vi "HPMT_View.vi"() -> ()   [LabVIEW 2016, in "HPMT_Views.lvlib"]
uses:
  HPMT_Views.lvlib
  Commands/Command Factory/Command Factory.lvclass
  User Events/User Events.lvclass
  User Events/User Events.lvclass/User Events.ctl
  Typedefs/CommandTypes.ctl
  Typedefs/StateTypes.ctl
  Typedefs/HPMT_Typedefs.lvlib
  Controller/Controller.lvclass
  Settings/Settings.lvclass
panel:
  in  "Tab Control":enum32{"Control"}(tab)
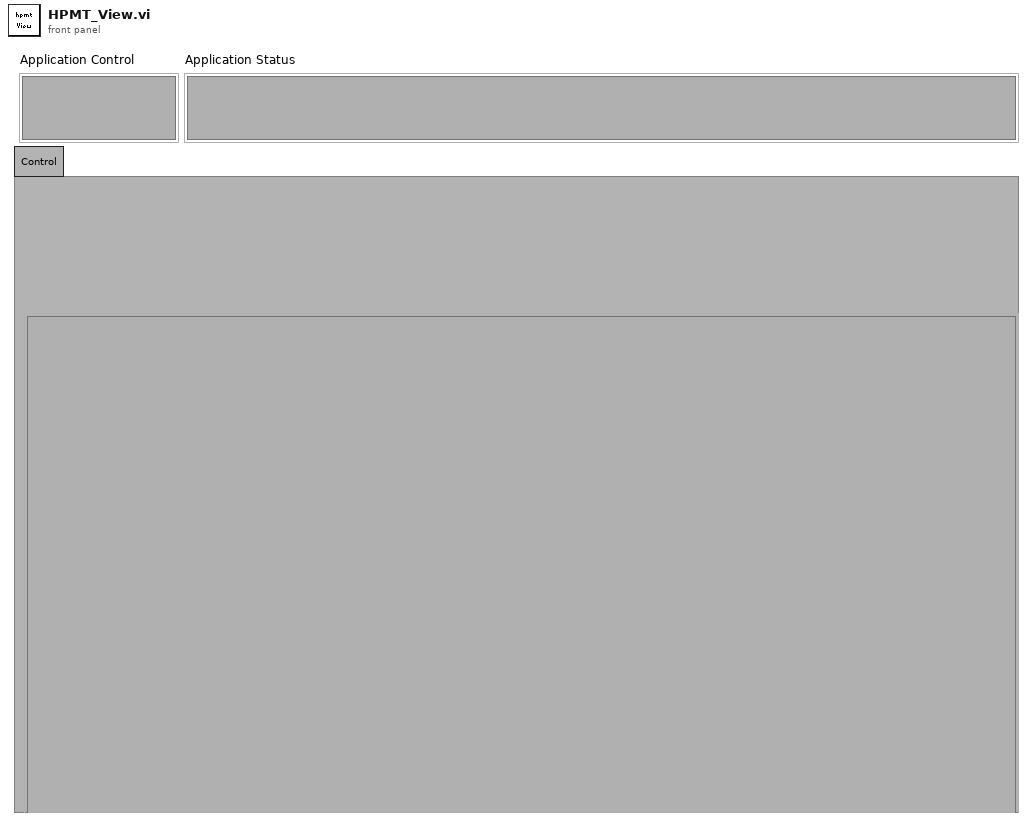
[diagram p1: front panel]
types:
  T1 = enum32{"invalid app kind", "Development System", "Run Time System", "Student Edition", "Embedded LabVIEW", "Evaluation", "Custom"}
  T2 = typedef "HPMT_Typedefs.lvlib/Publish Data Events.ctl" = cluster{"State":refnum<user-event>, "ErrorCode":refnum<user-event>, "Scan Progress":refnum<user-event>, "All Test Status":refnum<user-event>, "ActuatorData":refnum<user-event>, "Test Settings":refnum<user-event>, "Stop Constant Query":refnum<user-event>}
  T3 = typedef "HPMT_Typedefs.lvlib/Subscribe Data Events.ctl" = cluster{"Command":refnum<user-event>}
  T4 = cluster{"Event Registration Refnum":refnum<event-registration>, "Event Registration Refnum":refnum<event-registration>}
  T5 = typedef "HPMT_Typedefs.lvlib/CommandTypes.ctl" = enum16{"Start", "Enable", "Disable", "Standby", "Shutdown", "Update", "Stiffness", "Move Steps", "Constant Query", "Stop Constant Query"}
  T6 = typedef "HPMT_Typedefs.lvlib/StateTypes.ctl" = enum16{"Offline State", "Fault State", "Standby State", "Disabled State", "Enabled State", "Wait For User Input State", "Test Actuator State", "Manual State"}
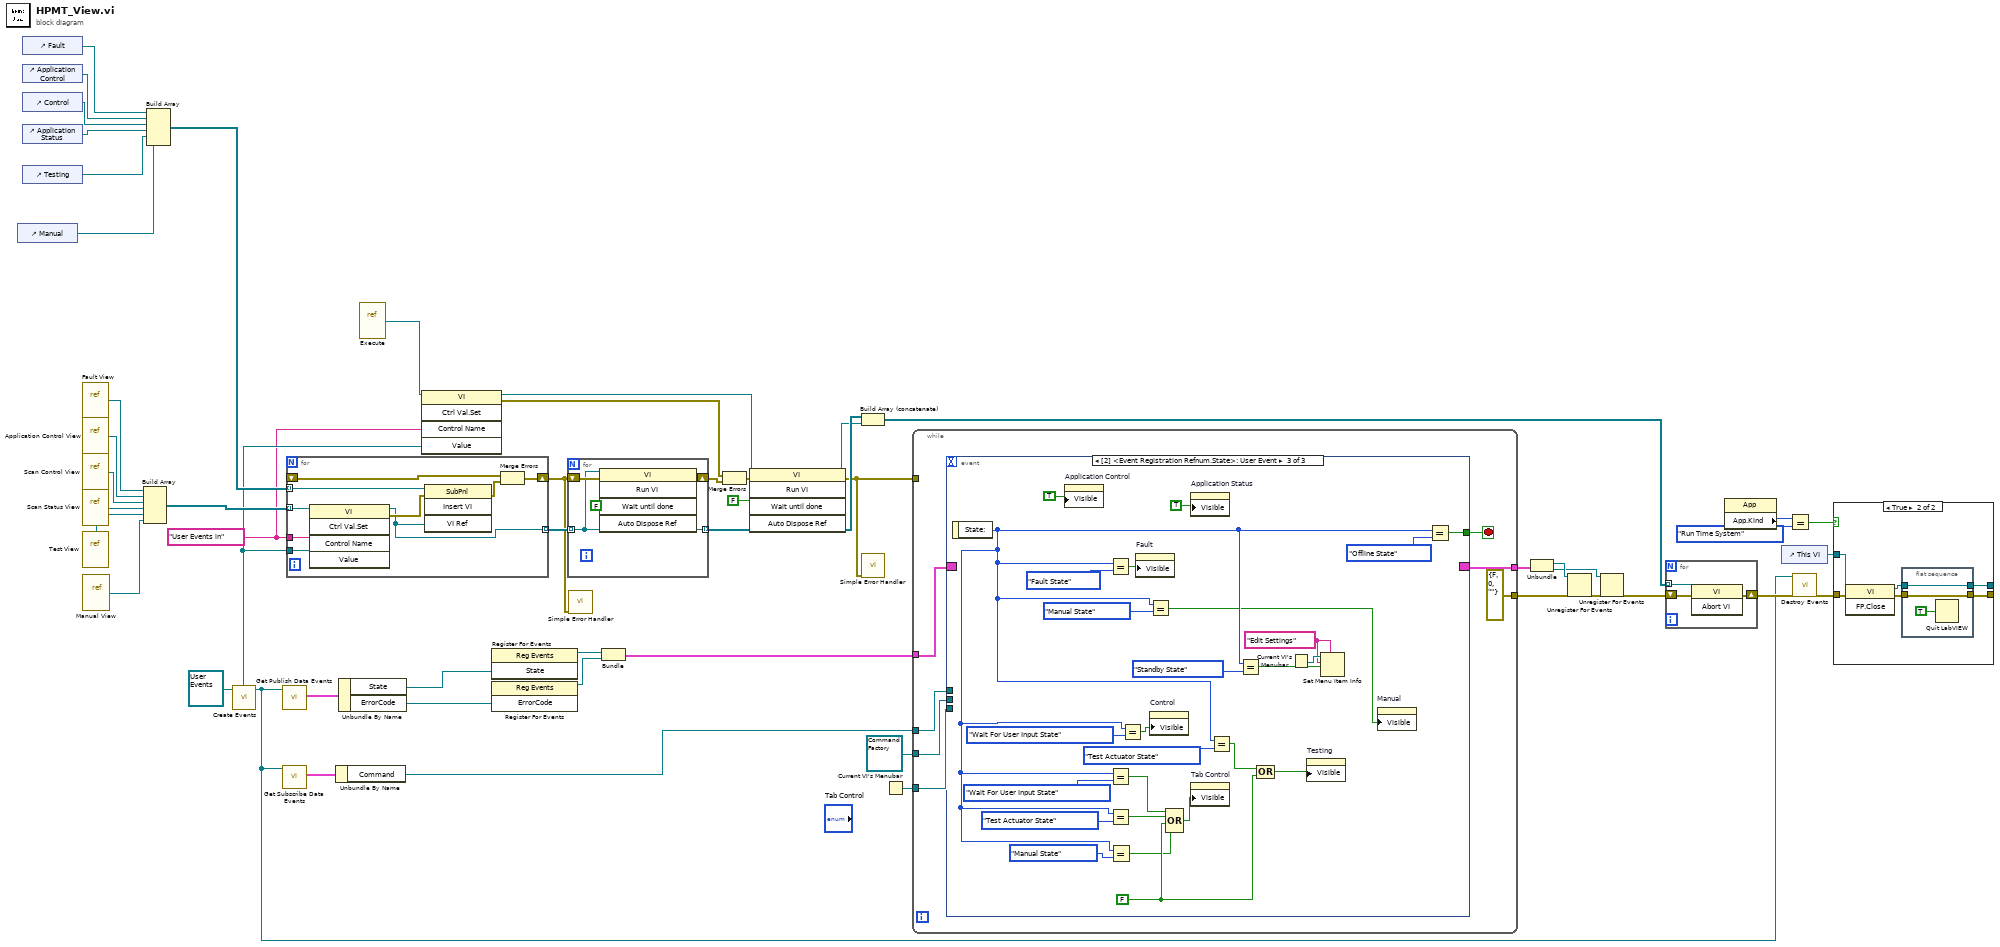
[diagram p0: block diagram]
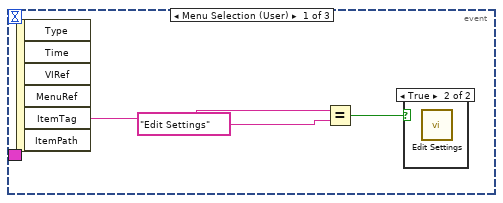
[diagram p3: hidden frame]
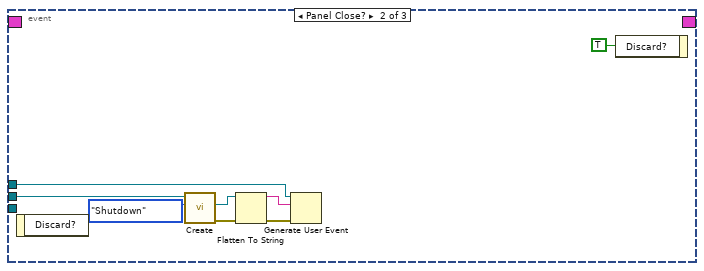
[diagram p5: hidden frame]
diagram:
  w21 = "User Events in" ("Control Name")
  n1 = control-ref of="Manual"() -> (w1:refnum<vi>)
  n2 = control-ref of="Fault"() -> (w11:refnum<vi>)
  n3 = control-ref of="Application Control"() -> (w10:refnum<vi>)
  n4 = control-ref of="Control"() -> (w9:refnum<vi>)
  n5 = control-ref of="Application Status"() -> (w8:refnum<vi>)
  n6 = control-ref of="Testing"() -> (w4:refnum<vi>)
  n7 = vi-ref "Fault View.vi"() -> (w26:refnum<vi>)
  n8 = vi-ref "Application Control View.vi"() -> (w7:refnum<vi>)
  n9 = vi-ref "Scan Control View.vi"() -> (w6:refnum<vi>)
  n10 = vi-ref "Scan Status View.vi"() -> (w12:refnum<vi>)
  n11 = vi-ref "Test View.vi"() -> (w3:refnum<vi>)
  n12 = vi-ref "Manual View.vi"() -> (w2:refnum<vi>)
  n13 = Build Array(w26, w7, w6, w12, w3, w2) -> (w24:refnum<vi>[])
  n14 = Build Array(w11, w10, w9, w8, w4, w1) -> (w25:refnum<vi>[])
  n15 = call "Create Events.vi"("UserEvents in"=refnum<class "User Events.lvclass"> refnum) -> ("UserEvents out"=w22:refnum<class "User Events.lvclass">)  [unwired: 9 in, 1 out]
  n16 = call "Get Publish Data Events.vi"("UserEvents in"=w22) -> ("Publish Data Events"=w46:T2)  [unwired: 9 in, 1 out]
  n17 = call "Get Subscribe Data Events.vi"("UserEvents in"=w22) -> ("Subscribe Data Events"=w44:T3)  [unwired: 9 in, 1 out]
  n18 = for {
    tunnel: w22 -> [w60]
    tunnel: w25 -> [w59] mode=indexing
    tunnel: w24 -> [w53] mode=indexing
    shift-right: [w58] -> w14
    shift-left: _ -> [w57]
    tunnel: [w52] -> w23 mode=indexing
    tunnel: w21 -> [w56]
    n19 = invoke class="VI" method="Ctrl Val.Set"(reference=w53, "Control Name"=w56, "Value"=w60) -> (reference out=w52:refnum<vi>, error out=w55:errorcluster)  [unwired: 2 in, 3 out]
    n20 = invoke on="Invoke Node" class="SubPnl" method="Insert VI"(reference=w59, error in=w55, "VI Ref"=w52) -> (error out=w54:errorcluster)  [unwired: 1 in, 3 out]
    n21 = Merge Errors(w57, w54) -> (w58:errorcluster)
  }
  n22 = Unbundle By Name(w44) -> ("Command"=w43:refnum<user-event>)
  n23 = Unbundle By Name(w46) -> ("State"=w42:refnum<user-event>, "ErrorCode"=w40:refnum<user-event>)
  n24 = vi-ref "Execute.vi"() -> (w37:refnum<vi>)
  n25 = invoke class="VI" method="Ctrl Val.Set"(reference=w37, "Control Name"=w21, "Value"=w22) -> (reference out=w36:refnum<vi>, error out=w18:errorcluster)  [unwired: 2 in, 3 out]
  n26 = register-events(w42) -> (reference out=w41:refnum<event-registration>)  [unwired: 2 in, 1 out]
  n27 = register-events(w40) -> (reference out=w39:refnum<event-registration>)  [unwired: 2 in, 1 out]
  n28 = for {
    shift-right: [w64] -> w20
    shift-left: w14 -> [w63]
    tunnel: w23 -> [w61] mode=indexing
    tunnel: [w61] -> w17 mode=indexing
    n29 = invoke class="VI" method="Run VI"(reference=w61, error in=w63, "Wait until done"=FALSE ("Wait Until Done")) -> (error out=w64:errorcluster)  [unwired: 2 in, 4 out]
  }
  n30 = call <vilib>:"Simple Error Handler.vi"("error in (no error)"=w14) -> ()  [unwired: 4 in, 5 out]
  n31 = Bundle("Event Registration Refnum"=w41, "Event Registration Refnum"=w39) -> (w34:T4)  [unwired: 1 in]
  n32 = Merge Errors(w18, w20) -> (w19:errorcluster)
  n33 = invoke class="VI" method="Run VI"(reference=w36, error in=w19, "Wait until done"=FALSE ("Wait Until Done")) -> (reference out=w16:refnum<vi>, error out=w13:errorcluster)  [unwired: 2 in, 3 out]
  n34 = Build Array (concatenate)(w17, w16) -> (w15:refnum<vi>[])
  n35 = call <vilib>:"Simple Error Handler.vi"("error in (no error)"=w13) -> ()  [unwired: 4 in, 5 out]
  n36 = Current VI's Menubar() -> (w47:refnum<k9>)
  n37 = while {
    tunnel: refnum<class "Command Factory.lvclass"> refnum ("CommandFactory.lvclass") -> [w68]
    tunnel: [errorcluster {"status"=FALSE, "code"=0, "source"=""} ("error out")] -> w35
    tunnel: w47 -> [w66]
    tunnel: w34 -> [w70]
    tunnel: w43 -> [w67]
    tunnel: [w65] -> w33
    tunnel: w13 -> [_]
    stop <- w69 stop-if-true
    n38 = event shown="[2] <Event Registration Refnum.State>: User Event" {
      selector: w70 -> [_ _ _]
      dyn-events: [_ _ _] -> w65
      timeout: _ -> [_ _ _]
      tunnel: [_ _ w107] -> w69
      tunnel: w68 -> [_ w79 _]
      tunnel: w67 -> [_ w76 _]
      tunnel: w66 -> [_ _ _]
      event Menu Selection (User) {
        n39 = event-data() -> ("ItemTag"=w72:string)  [unwired: 1 in, 5 out]
        n40 = Equal?(x=w72, y="Edit Settings") -> (x = y?=w74:bool)
        n41 = case shown="True" w74 {
          frame False {
          }
          frame True {
            n42 = call "Edit Settings.vi"() -> ()  [unwired: 10 in, 2 out]
          }
        }
      }
      event Panel Close? {
        n43 = event-data() -> ()  [unwired: 1 in, 1 out]
        n44 = call-dynamic "Create.vi"("Command Types"=CommandTypes."Shutdown" ("Command"), "Command Factory in"=w79) -> ("error out"=w82:errorcluster, "Command"=w81:refnum<class "Command.lvclass">)  [unwired: 7 in, 1 out]
        n45 = Flatten To String(anything=w81, error in (no error)=w82) -> (data string=w77:string, error out=w78:errorcluster)  [unwired: 2 in, 1 out]
        n46 = Generate User Event(user event=w76, event data cluster=w77, error in=w78) -> ()  [unwired: 1 in, 2 out]
        n47 = event-data("Discard?"=TRUE) -> ()  [unwired: 1 in, 1 out]
      }
      event User Event {
        w91 = FALSE
        w99 = "Edit Settings" ("menu tag")
        n48 = event-data() -> ("State:"=w84:T6)  [unwired: 1 in]
        n49 = property on="Application Control" class="SubPnl"("Visible"=TRUE) -> ()  [unwired: 2 in, 2 out]
        n50 = Equal?(x=w84, y=StateTypes."Fault State") -> (x = y?=w104:bool)
        n51 = Equal?(x=w84, y=StateTypes."Wait For User Input State") -> (x = y?=w94:bool)
        n52 = Equal?(x=w84, y=StateTypes."Test Actuator State") -> (x = y?=w88:bool)
        n53 = Equal?(x=w84, y=StateTypes."Manual State") -> (x = y?=w86:bool)
        n54 = Equal?(x=w84, y=StateTypes."Wait For User Input State") -> (x = y?=w89:bool)
        n55 = property on="Fault" class="SubPnl"("Visible"=w104) -> ()  [unwired: 2 in, 2 out]
        n56 = Equal?(x=w84, y=StateTypes."Manual State") -> (x = y?=w83:bool)
        n57 = property on="Control" class="SubPnl"("Visible"=w89) -> ()  [unwired: 2 in, 2 out]
        n58 = Compound Arithmetic op=OR(w94, w88, w91, w86) -> (w93:bool)
        n59 = property on="Application Status" class="SubPnl"("Visible"=TRUE) -> ()  [unwired: 2 in, 2 out]
        n60 = property on="Tab Control" class="TabCtl (strict)"("Visible"=w93) -> ()  [unwired: 2 in, 2 out]
        n61 = Equal?(x=w84, y=StateTypes."Test Actuator State") -> (x = y?=w92:bool)
        n62 = Equal?(x=w84, y=StateTypes."Standby State") -> (x = y?=w100:bool)
        n63 = Compound Arithmetic op=OR(w92, w91) -> (w90:bool)
        n64 = Current VI's Menubar() -> (w101:refnum<k9>)
        n65 = property on="Testing" class="SubPnl"("Visible"=w90) -> ()  [unwired: 2 in, 2 out]
        n66 = Set Menu Item Info(7:w99, 9:w100, 10:w99, 11:w101) -> ()  [unwired: 3 in, 2 out]
        n67 = property on="Manual" class="SubPnl"("Visible"=w83) -> ()  [unwired: 2 in, 2 out]
        n68 = Equal?(x=w84, y=StateTypes."Offline State") -> (x = y?=w107:bool)
      }
    }
  }
  n69 = Unbundle(w33) -> ("Event Registration Refnum"=w32:refnum<event-registration>, "Event Registration Refnum"=w30:refnum<event-registration>)
  n70 = Unregister For Events(event registration refnum=w32, error in=w35) -> (error out=w31:errorcluster)
  n71 = Unregister For Events(event registration refnum=w30, error in=w31) -> (error out=w5:errorcluster)
  n72 = for {
    tunnel: w15 -> [w109] mode=indexing
    shift-right: [w110] -> w29
    shift-left: w5 -> [w111]
    n73 = invoke class="VI" method="Abort VI"(reference=w109, error in=w111) -> (error out=w110:errorcluster)  [unwired: 1 in, 2 out]
  }
  n74 = property class="App"() -> ("App.Kind"=w51:T1)  [unwired: 2 in, 2 out]
  n75 = control-ref of="This VI"() -> (w28:refnum<vi>)
  n76 = Equal?(x=w51, y=T1."Run Time System") -> (x = y?=w49:bool)
  n77 = call "Destroy Events.vi"("error in (no error)"=w29, "UserEvents in"=w22) -> ("error out"=w27:errorcluster)  [unwired: 8 in, 1 out]
  n78 = case shown="True" w49 {
    tunnel: w28 -> [w113 w119]
    tunnel: w27 -> [w112 w118]
    tunnel: [w113 w116] -> _
    tunnel: [w112 w114] -> _
    frame False {
    }
    frame True {
      n79 = invoke class="VI" method="FP.Close"(reference=w119, error in=w118) -> (reference out=w115:refnum<vi>, error out=w117:errorcluster)  [unwired: 1 in, 1 out]
      n80 = flat-sequence {
        tunnel: w117 -> [w120]
        tunnel: [w121] -> w116
        tunnel: w115 -> [w121]
        tunnel: [w120] -> w114
        frame #0 {
          n81 = Quit LabVIEW(quit? (T)=TRUE) -> ()
        }
      }
    }
  }
